vi "CRYPIC Step SHowHide.vi"(7 "sAction":string, 10 "VIRef":refnum<vi>) -> ()   [LabVIEW 2013]
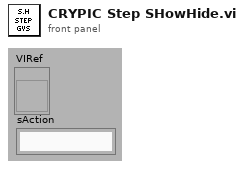
[diagram p1: front panel]
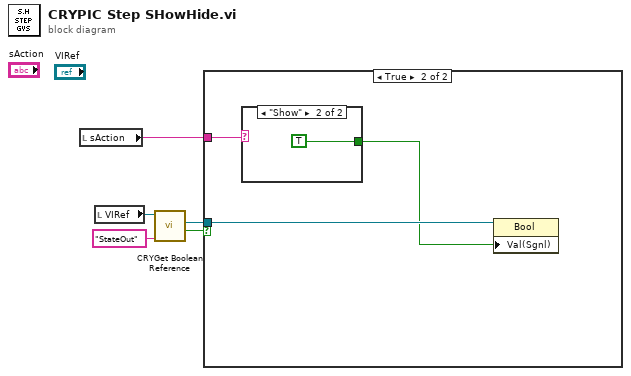
[diagram p0: block diagram]
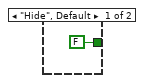
[diagram p3: hidden frame]
diagram:
  n1 = local read "sAction"() -> (w1:string)
  n2 = local read "VIRef"() -> (w5:refnum<vi>)
  n3 = call "CRYGet Boolean Reference.vi"("Label Name"="StateOut", "VI Refnum"=w5) -> ("Exist?"=w3:bool, "Boolean Ref"=w2:refnum<vi>)  [unwired: 7 in, 1 out]
  n4 = case shown="True" w3 {
    tunnel: w2 -> [_ w7]
    tunnel: w1 -> [_ w8]
    frame False {
    }
    frame True {
      n5 = case shown="\"Show\"" w8 {
        tunnel: [FALSE TRUE] -> w6
        frame "Hide", Default {
        }
        frame "Show" {
        }
      }
      n6 = property class="Bool"(reference=w7, "Val(Sgnl)"=w6) -> ()  [unwired: 1 in, 2 out]
    }
  }
